vi "getFPGA.vi"(11 "ModbusSubnetCTxDataFIFO in":refnum<class "ModbusSubnetCTxDataFIFO.lvclass">) -> (2 "FPGA":refnum<class "FPGA.lvclass">, 3 "ModbusSubnetCTxDataFIFO out":refnum<class "ModbusSubnetCTxDataFIFO.lvclass">)   [LabVIEW 2016, in "ModbusSubnetCTxDataFIFO.lvclass"]
uses:
  ModbusSubnetCTxDataFIFO.lvclass
  FPGA/FPGA.lvclass
  ModbusSubnetCTxDataFIFO.lvclass/ModbusSubnetCTxDataFIFO.ctl
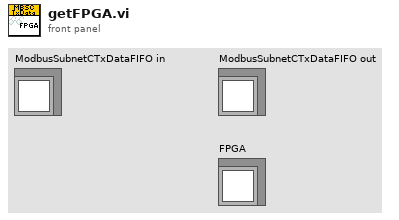
[diagram p1: front panel]
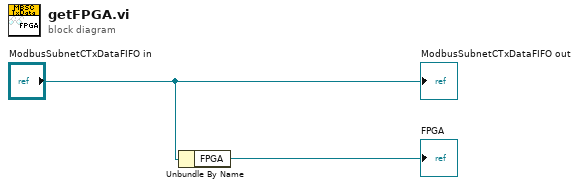
[diagram p0: block diagram]
diagram:
  n1 = Unbundle By Name("ModbusSubnetCTxDataFIFO in") -> ("FPGA"=→"FPGA":refnum<class "FPGA.lvclass">)
  "ModbusSubnetCTxDataFIFO out" <- "ModbusSubnetCTxDataFIFO in"
